vi "Get Column Config.vi"(8 "error in (no error)":errorcluster, 11 "By-Value Column in":refnum<class "By-Value Column.lvclass">) -> (0 "error out":errorcluster, 2 "Column Configuration":refnum<class "Column Configuration.lvclass">, 3 "By-Value Column out":refnum<class "By-Value Column.lvclass">)   [LabVIEW 2020, in "Basic Columns.lvlib" / "By-Value Column.lvclass"]
uses:
  By-Value Column.lvclass
  Column Interface/Column Configuration Interface Class/Column Configuration.lvclass
  By-Value Column.lvclass/By-Value Column.ctl
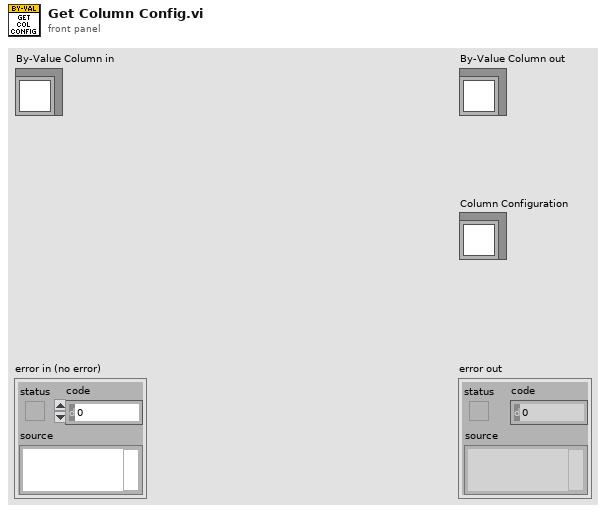
[diagram p1: front panel]
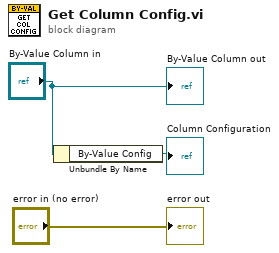
[diagram p0: block diagram]
diagram:
  n1 = Unbundle By Name("By-Value Column in") -> ("By-Value Config"=→"Column Configuration":refnum<class "Column Configuration.lvclass">)
  "error out" <- "error in (no error)"
  "By-Value Column out" <- "By-Value Column in"
